vi "INTERLOCK SETTING.vi"() -> ()   [LabVIEW 2017]
uses:
  <vilib>/addons/database/Connection.llb/DB Tools Open Connec (Path).vi
  <vilib>/addons/database/NI_Database_API.lvlib
panel:
  in  "table":string[][](table)
  in  "EXIT":bool
  in  "SAVE":bool
  # "PARAMETERS VALUE"
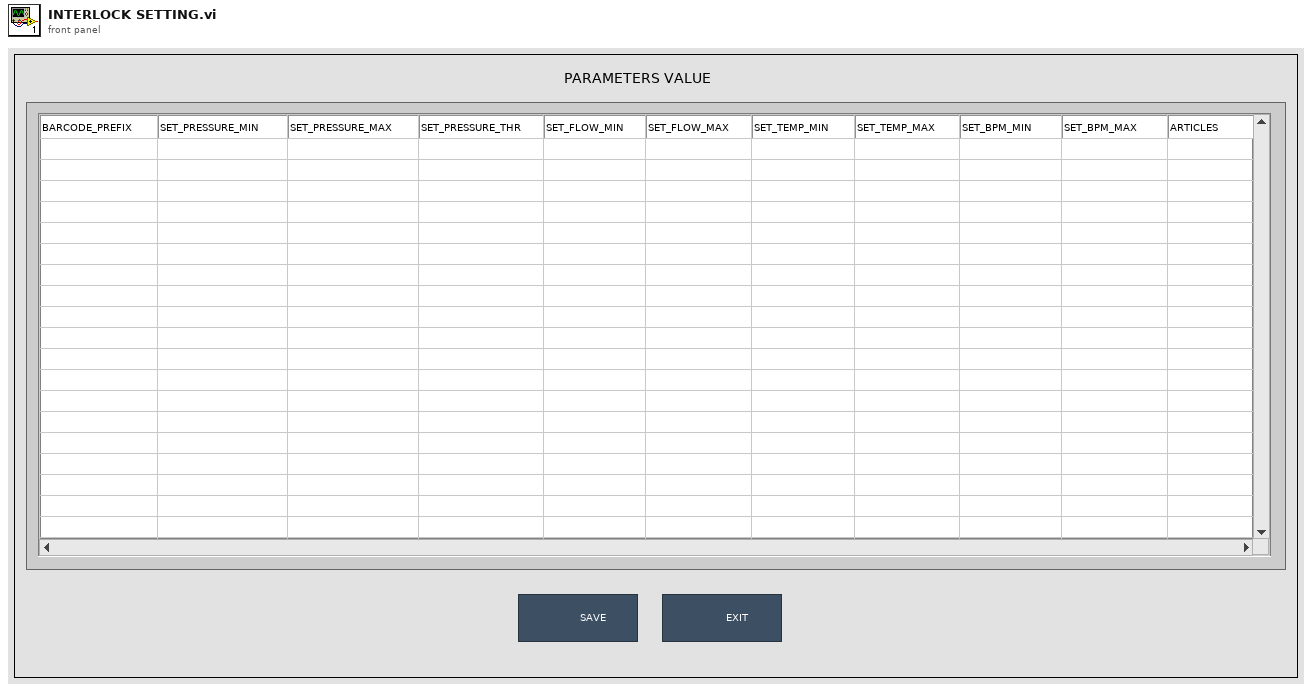
[diagram p1: front panel]
types:
  T1 = typedef "NI_Database_API.lvlib/Conn ObjectReference.ctl" = refnum<k1>
  T2 = cluster{"table":string[], "table":string[], "table":string[], "table":string[], "table":string[], "table":string[], "table":string[], "table":string[], "table":string[], "table":string[], "table":string[], "table":string[]}
  T3 = enum32{"invalid app kind", "Development System", "Run Time System", "Student Edition", "Embedded LabVIEW", "Evaluation", "Custom"}
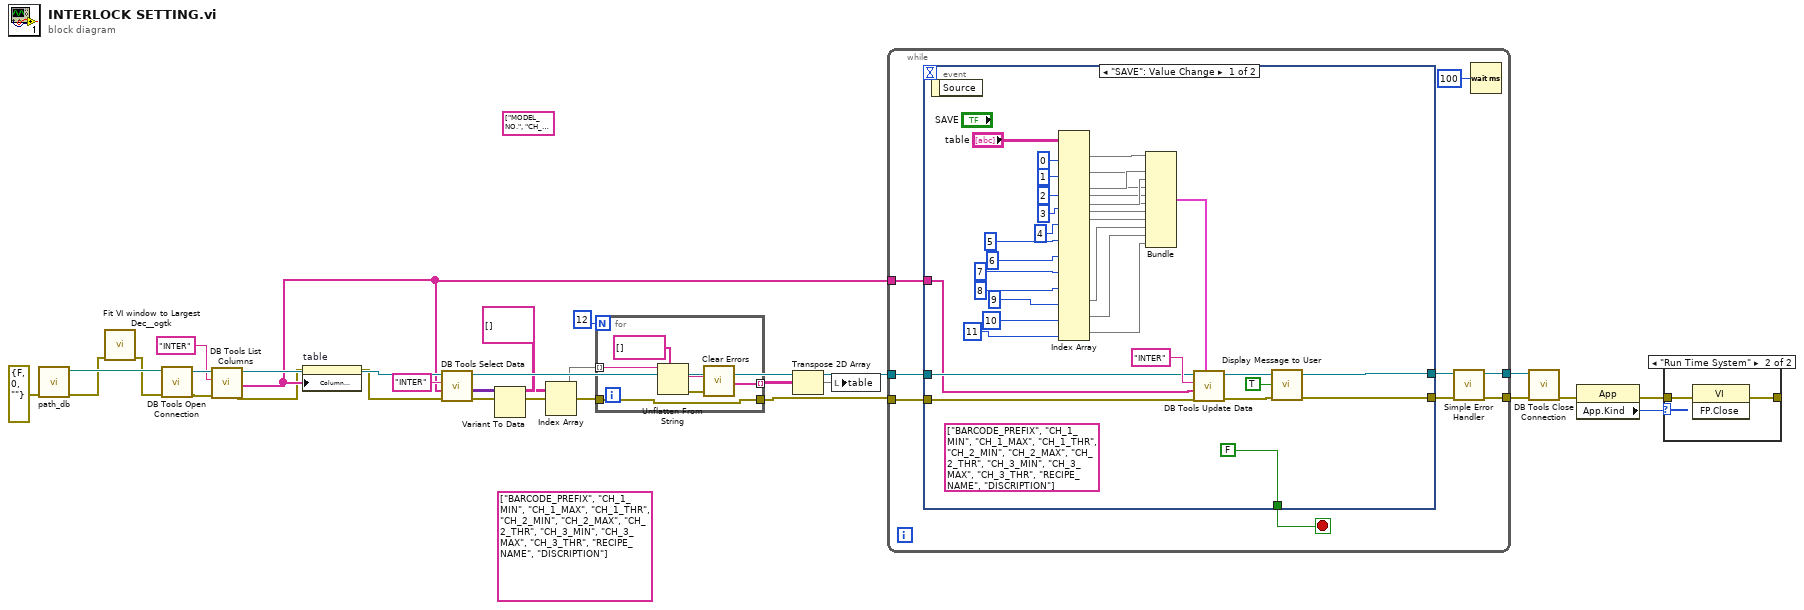
[diagram p0: block diagram]
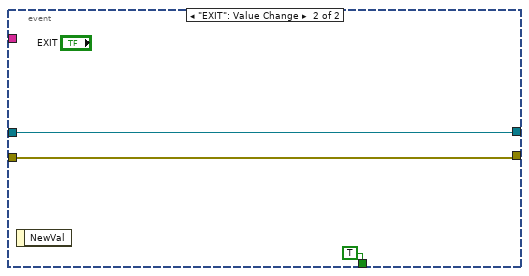
[diagram p3: hidden frame]
diagram:
  (unwired) string[] ["MODEL_NO.", "CH_1_MIN", "CH_1_MAX", "CH_1_THR", "CH_2_MIN", "CH_2_MAX", "CH_2_THR", "CH_3_MIN", "CH_3_MAX", "CH_3_THR", "RECIPE NAME", "DESCRIPTION"] ("Column Header Strings[]")
  (unwired) string[] ["BARCODE_PREFIX", "CH_1_MIN", "CH_1_MAX", "CH_1_THR", "CH_2_MIN", "CH_2_MAX", "CH_2_THR", "CH_3_MIN", "CH_3_MAX", "CH_3_THR", "RECIPE_NAME", "DISCRIPTION"]
  n1 = call "path_db.vi"("error in"=errorcluster {"status"=FALSE, "code"=0, "source"=""}) -> ("error out"=w10:errorcluster, "resulting string"=w16:path)  [unwired: 9 in]
  n2 = call <userlib>:"Fit VI window to Largest Dec__ogtk.vi"("error in (no error)"=w10) -> ("error out"=w9:errorcluster)  [unwired: 5 in, 1 out]
  n3 = call-poly <vilib>:"DB Tools Open Connection.vi"("error in (no error)"=w9, "connection information"=w16) -> ("error out"=w7:errorcluster, "connection reference"=w6:T1)  [unwired: 6 in]
  n4 = call <vilib>:"DB Tools List Columns.vi"("error in (no error)"=w7, "table"="INTER", "connection reference"=w6) -> ("error out"=w2:errorcluster, "columns"=w3:string[], "connection reference out"=w5:T1)  [unwired: 1 in, 1 out]
  n5 = property on="table" class="Tbl (strict)"(error in=w2, "Column Headers[]"=w3) -> (error out=w1:errorcluster)  [unwired: 1 in, 1 out]
  n6 = call <vilib>:"DB Tools Select Data.vi"("error in (no error)"=w1, "columns"=w3, "table"="INTER", "connection reference"=w5) -> ("error out"=w12:errorcluster, "data"=w19:variant[][], "connection reference out"=w22:T1)  [unwired: 2 in]
  n7 = Variant To Data(type=string[][] [], Variant=w19) -> (data=w18:string[][])  [unwired: 1 in, 1 out]
  n8 = Index Array(array=w18) -> (element=w14:string[])  [unwired: 2 in]
  n9 = for {
    N: 12 -> [_]
    tunnel: w14 -> [w31] mode=indexing
    tunnel: [w29] -> w13 mode=indexing
    tunnel: w12 -> [w28]
    tunnel: [w28] -> w11
    n10 = Unflatten From String(type=string[] [], binary string=w31) -> (value=w29:string[], error out=w32:errorcluster)  [unwired: 3 in, 1 out]
    n11 = call <vilib>:"Clear Errors.vi"("error in (no error)"=w32) -> ()  [unwired: 5 in, 2 out]
  }
  n12 = Transpose 2D Array(2D array=w13) -> (transposed array=w17:string[][])
  n13 = local write "table"(w17) -> ()
  n14 = while {
    tunnel: w11 -> [w39]
    tunnel: w22 -> [w38]
    tunnel: [w37] -> w27
    tunnel: [w35] -> w26
    tunnel: w3 -> [w33]
    stop <- w40 stop-if-true
    n15 = event shown="[0] \"SAVE\": Value Change" {
      selector: _ -> [_ _]
      dyn-events: _ -> [_ _]
      timeout: _ -> [_ _]
      tunnel: [FALSE TRUE] -> w40
      tunnel: w39 -> [w73 w76]
      tunnel: w38 -> [w72 w77]
      tunnel: [w71 w77] -> w37
      tunnel: [w47 w76] -> w36
      tunnel: w33 -> [w43 _]
      event "SAVE": Value Change {
        (unwired) string[] ["BARCODE_PREFIX", "CH_1_MIN", "CH_1_MAX", "CH_1_THR", "CH_2_MIN", "CH_2_MAX", "CH_2_THR", "CH_3_MIN", "CH_3_MAX", "CH_3_THR", "RECIPE_NAME", "DISCRIPTION"]
        n16 = event-data() -> ()  [unwired: 1 in, 1 out]
        n17 = Index Array(array="table", index (col) #1=0 ("disabled index (col)"), index (col) #2=1 ("index (col)"), index (col) #3=2 ("index (col)"), index (col) #4=3 ("index (col)"), index (col) #5=4 ("index (col)"), index (col) #6=5 ("index (col)"), index (col) #7=6 ("index (col)"), index (col) #8=7 ("index (col)"), index (col) #9=8 ("index (col)"), index (col) #10=9 ("index (col)"), index (col) #11=10 ("index (col)"), index (col) #12=11 ("index (col)")) -> (element #1=w65:string[], element #2=w62:string[], element #3=w63:string[], element #4=w64:string[], element #5=w54:string[], element #6=w53:string[], element #7=w52:string[], element #8=w51:string[], element #9=w50:string[], element #10=w49:string[], element #11=w42:string[], element #12=w41:string[])  [unwired: 12 in]
        n18 = Bundle("table"=w65, "table"=w62, "table"=w63, "table"=w64, "table"=w54, "table"=w53, "table"=w52, "table"=w51, "table"=w50, "table"=w49, "table"=w42, "table"=w41) -> (w61:T2)  [unwired: 1 in]
        n19 = call <vilib>:"DB Tools Update Data.vi"("data"=w61, "error in (no error)"=w73, "columns"=w43, "table"="INTER", "connection reference"=w72) -> ("error out"=w48:errorcluster, "connection reference out"=w71:T1)  [unwired: 5 in]
        n20 = call "Display Message to User"("error in (no error)"=w48, "Enable"=TRUE) -> ("error out"=w47:errorcluster)  [unwired: 8 in, 1 out]
      }
      event "EXIT": Value Change {
        n21 = event-data() -> ()  [unwired: 1 in, 1 out]
      }
    }
    n22 = call <vilib>:"Simple Error Handler.vi"("error in (no error)"=w36) -> ("error out"=w35:errorcluster)  [unwired: 4 in, 4 out]
    n23 = Wait (ms)(milliseconds to wait=u32 100) -> ()  [unwired: 1 out]
  }
  n24 = call <vilib>:"DB Tools Close Connection.vi"("error in (no error)"=w26, "connection reference"=w27) -> ("error out"=w23:errorcluster)  [unwired: 5 in]
  n25 = property class="App"(error in=w23) -> (error out=w24:errorcluster, "App.Kind"=w25:T3)  [unwired: 1 in, 1 out]
  n26 = case shown="\"Run Time System\"" w25 {
    tunnel: w24 -> [w79 w81]
    tunnel: [w79 w80] -> _
    frame Default {
    }
    frame "Run Time System" {
      n27 = invoke class="VI" method="FP.Close"(error in=w81) -> (error out=w80:errorcluster)  [unwired: 2 in, 2 out]
    }
  }
